vi "DAQmx Read (Digital Wfm 1Chan NSamp Duration).vi"(0 "task/channels in":refnum<k21>, 7 "duration":dbl=1.0, 9 "timeout":dbl=10.0 format="%0.2f", 11 "error in":errorcluster) -> (4 "task out":refnum<k21>, 6 "data":digitalwaveform(waveform)={"t0"=timestamp(0 s since 1904-01-01), "dt"=0.0, "Y"={"transitions"=[], "data"=[]}, "error"={"status"=FALSE, "code"=37421928, "source"=""}}, 15 "error out":errorcluster)   [LabVIEW 2018]
uses:
  nilvaiu.dll
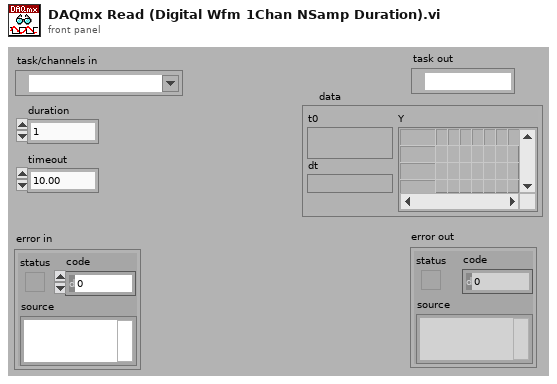
[diagram p1: front panel]
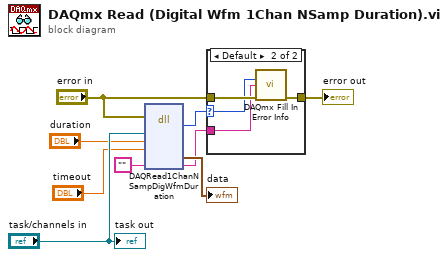
[diagram p0: block diagram]
diagram:
  n1 = dll-call lib="nilvaiu.*" fn="DAQRead1ChanNSampDigWfmDuration"(error in="error in", "taskID"="task/channels in", "duration"="duration", "timeout"="timeout", "extendedErrorInfo"="") -> ("return type"=w3:i32, "data"=→"data":digitalwaveform, "extendedErrorInfo"=w1:string)  [unwired: 4 in, 4 out]
  n2 = case shown="Default" w3 {
    selector: w3 -> [_ w12]
    tunnel: "error in" -> [w10 w14]
    tunnel: [w10 w13] -> w8
    tunnel: w1 -> [_ w11]
    frame 0 {
    }
    frame Default {
      n3 = call "DAQmx Fill In Error Info.vi"("status code"=w12, "extended error info"=w11, "error in"=w14) -> ("error out"=w13:errorcluster)  [unwired: 1 in, 11 out]
    }
  }
  "error out" <- w8
  "task out" <- "task/channels in"
